vi "Data_get.vi"() -> ()   [LabVIEW 2009]
uses:
  <vilib>/Analysis/2dsp.llb/Real FFT.vi
  <vilib>/Analysis/NI_AALPro.lvlib
panel:
  in  "ps/point":T1(ring)
  in  "ns/div":T2(ring)
  out "Current sweep":u32=1 min=1 max=1000 step=1
  in  "Ext":string="ccd"
  out "Number":string
  in  "Name":string="trace"
  in  "Folder":path
  in  "#Sweeps":u32=1 min=1 max=1000 step=1
  in  "Ampl. (dBm)":dbl min=-135.0 max=30.0 step=0.5 format="%#_8g"
  in  "f (MHz)":dbl=0.0003 min=0.00025 max=67.0 step=1e-06 format="%#.12f"
  in  "Start":bool
  in  "Quit":bool
  in  "E8257D VISA Port":refnum<visa-resource-name>="GPIB0::1::INSTR"
  out "read time (ms)":u32
  out "#points":u32
  out "Busy":bool
  in  "Repetition rate (Hz)":ext=2.5
  in  "Chirp start (MHz)":ext=2.5
  in  "Filter up to (MHz)":ext=2.5
  in  "Amount of averagings":u32=10
  out "Data":dbl[](array[numeric])
  out "XY Graph 5":cluster{ext[], dbl[]}(graph)
  out "FFT (Im)":dbl[](array[numeric])
  out "FFT (Re)":dbl[](array[numeric])
  out "Final array":ext[][](array[numeric])
  out "size(s)":i32
  out "Oscilloscope Data":dbl[](array[numeric])
  in  "Channel Number":u16=1
  out "Oscilloscope graph":dbl[](graph)
  in  "Stop":bool
  in  "TDS VISA Port":refnum<visa-resource-name>="GPIB0::1::INSTR"
  # "TDS6000"
  # "E8257D"
  # "Control"
  # "File Storage"
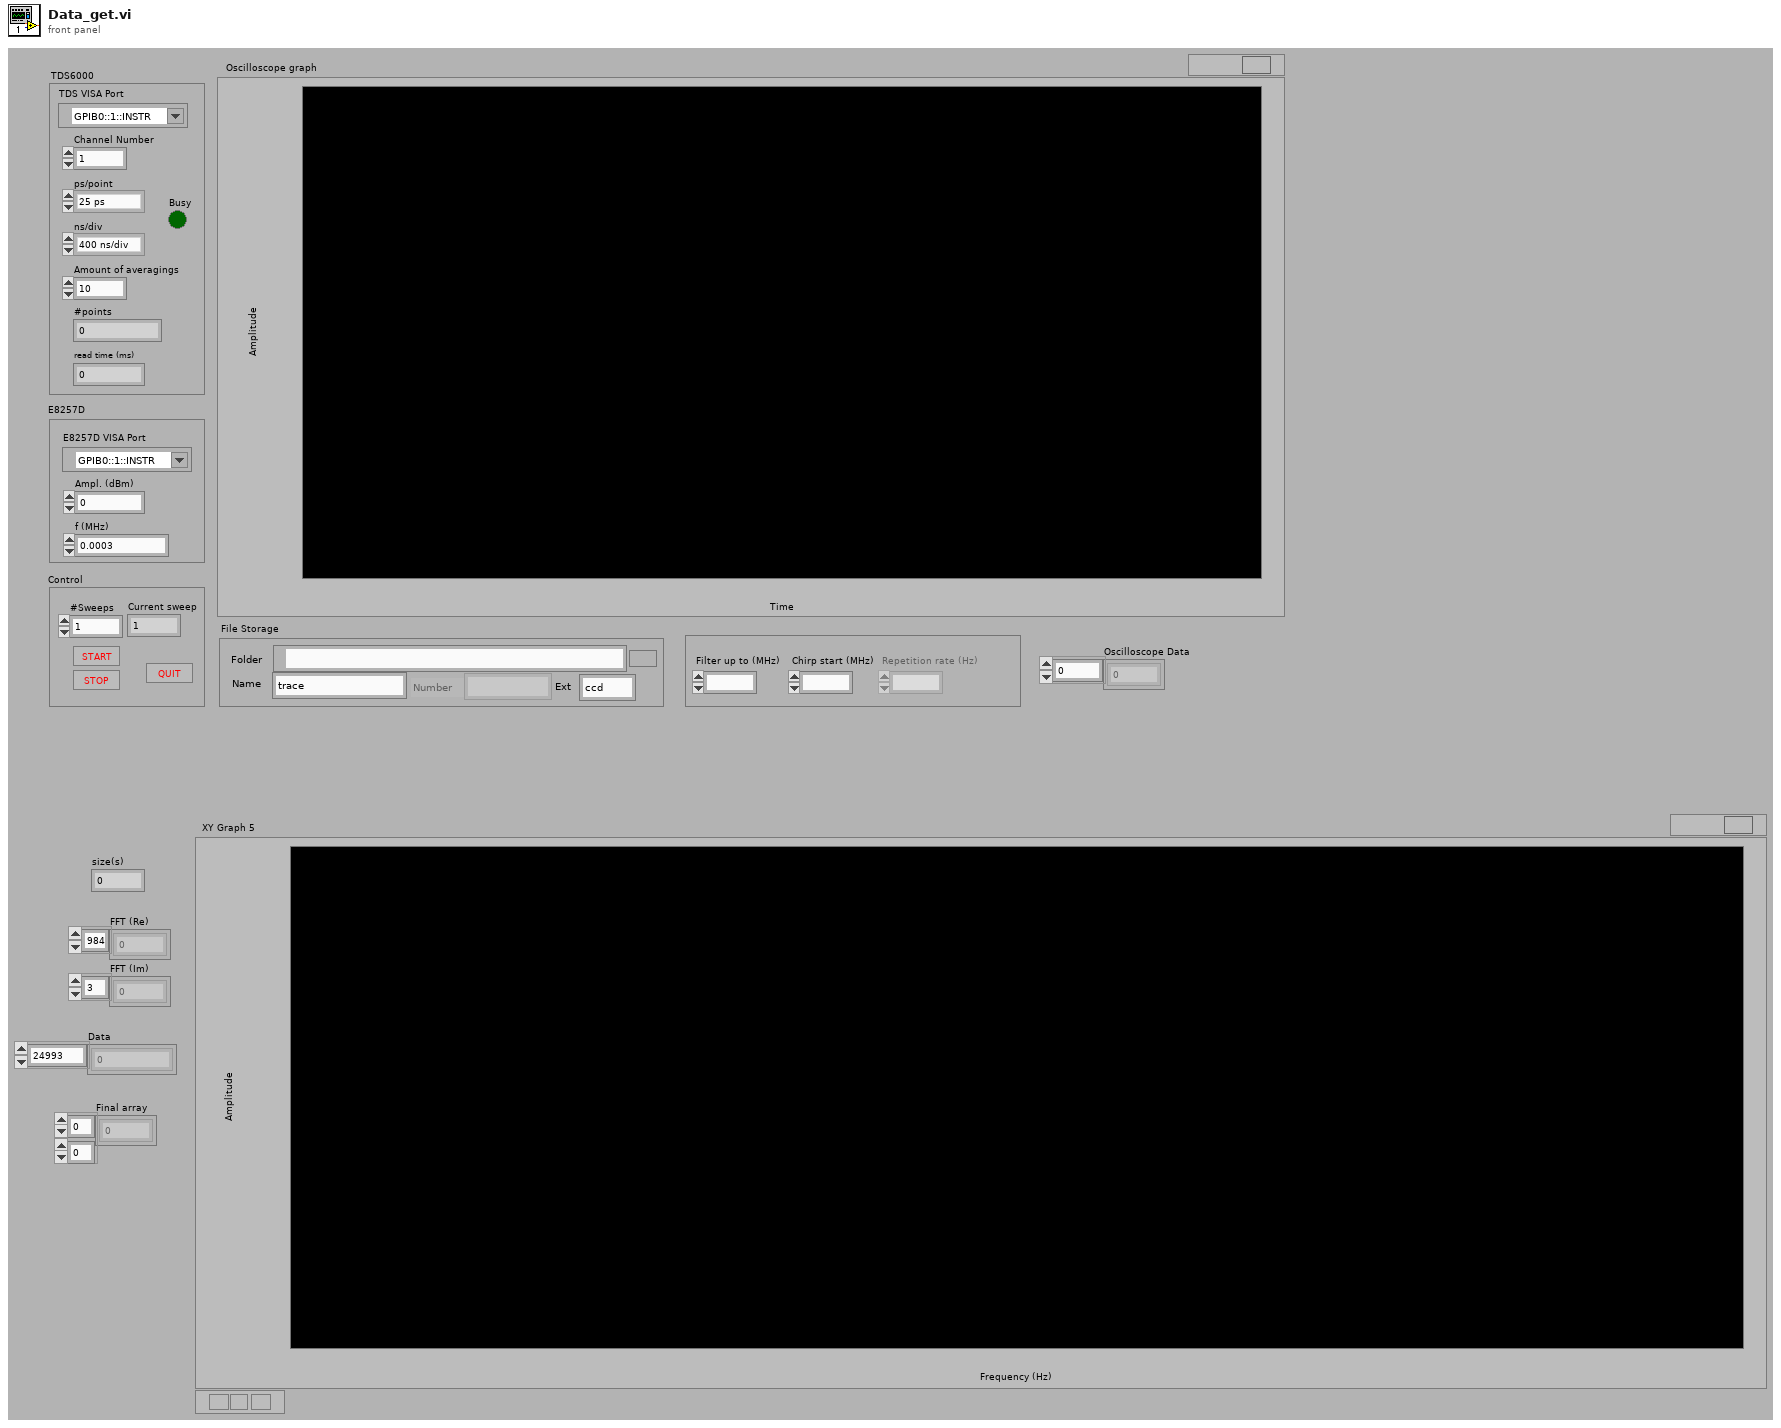
[diagram p1: front panel]
types:
  T1 = enum16{"25 ps", "50 ps", "100 ps", "200 ps", "400 ps", "800 ps", "2 ns"}
  T2 = enum16{"400 ns/div", "1 us/div", "2 us/div", "4 us/div", "10 us/div", "20 us/div"}
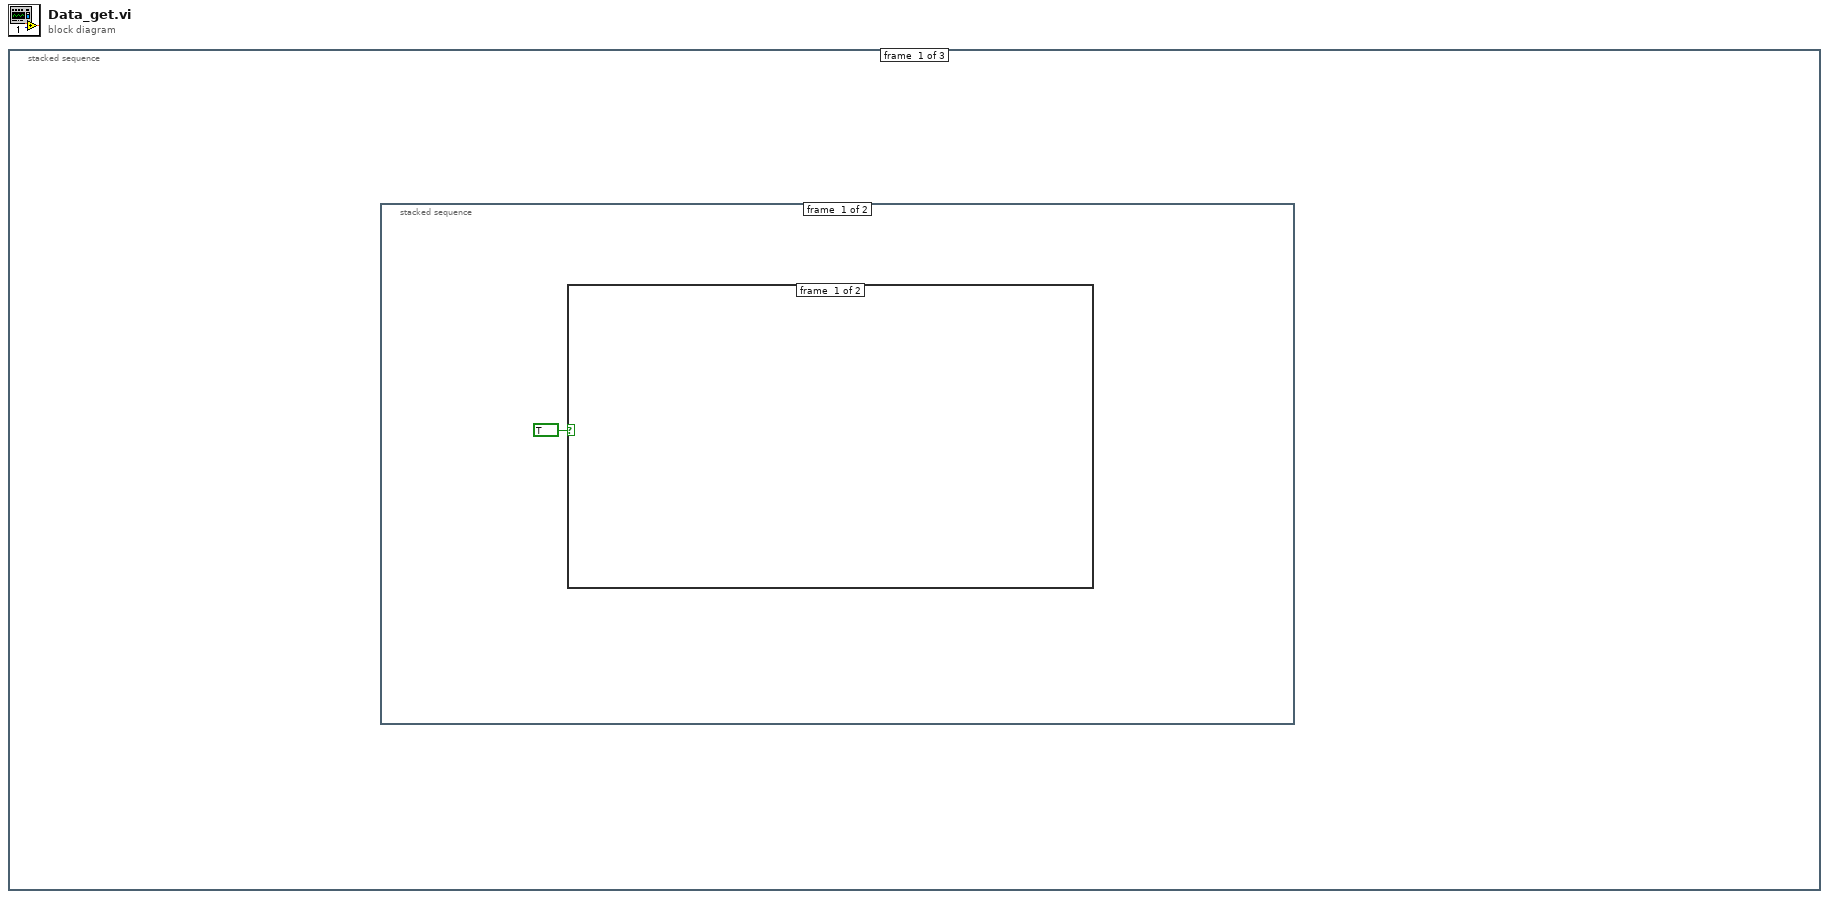
[diagram p0: block diagram]
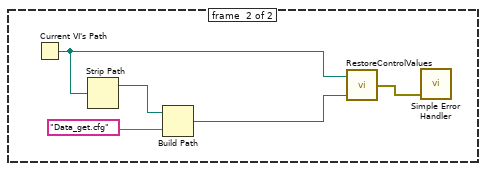
[diagram p2: hidden frame]
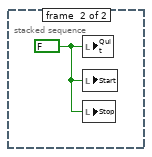
[diagram p3: hidden frame]
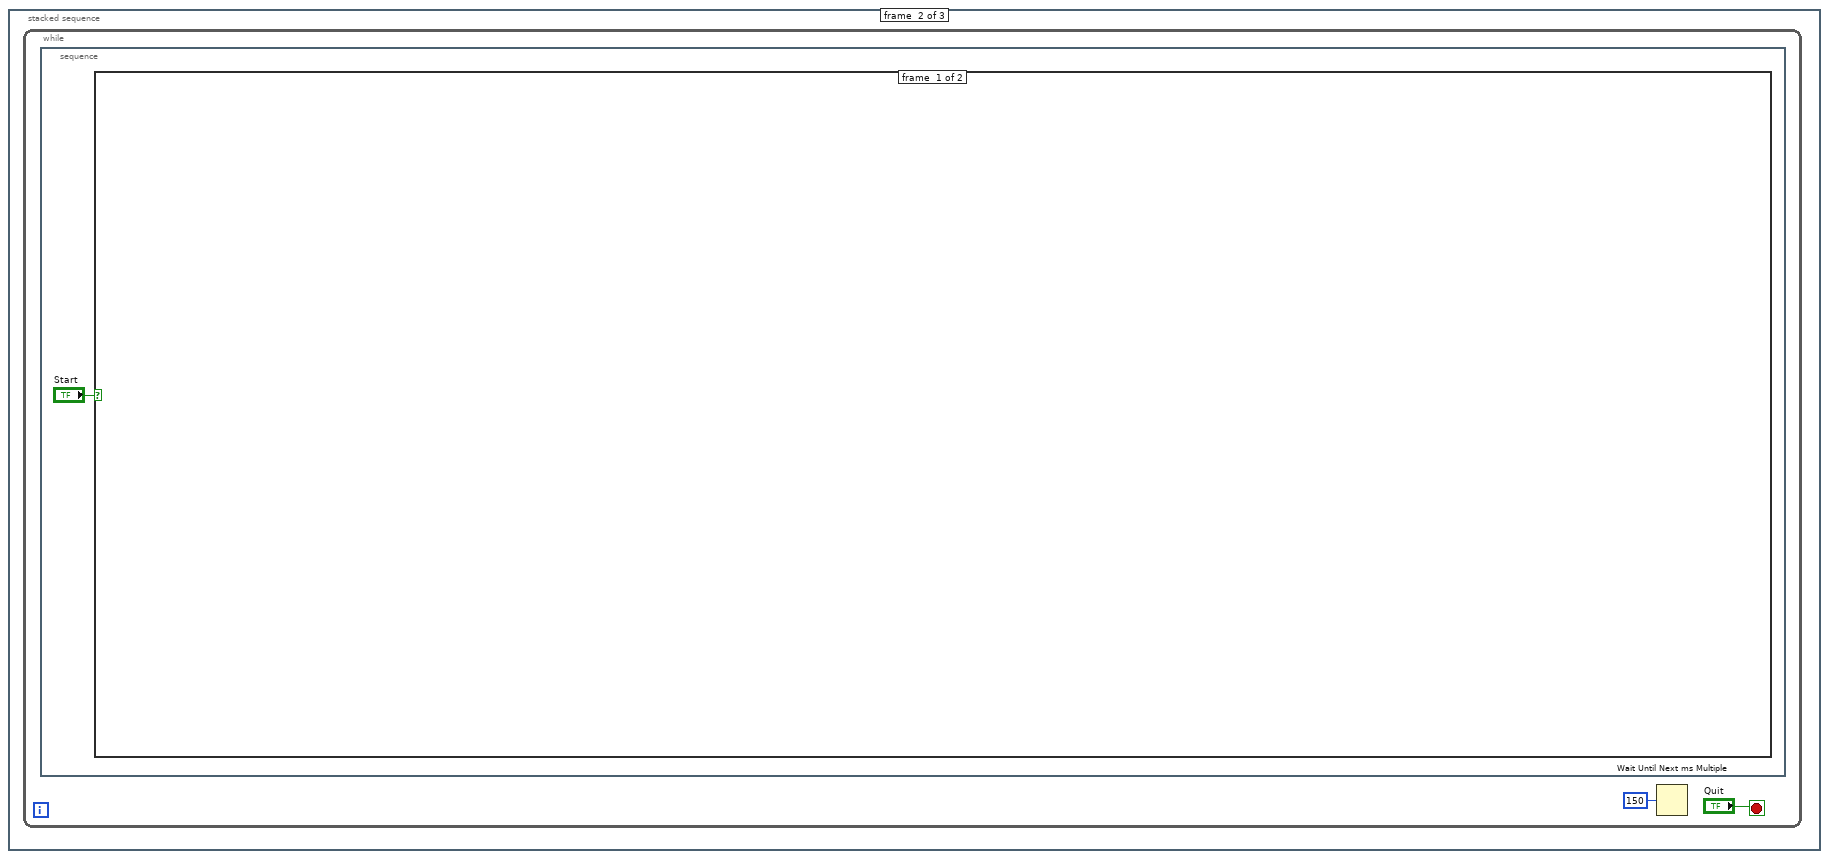
[diagram p4: hidden frame]
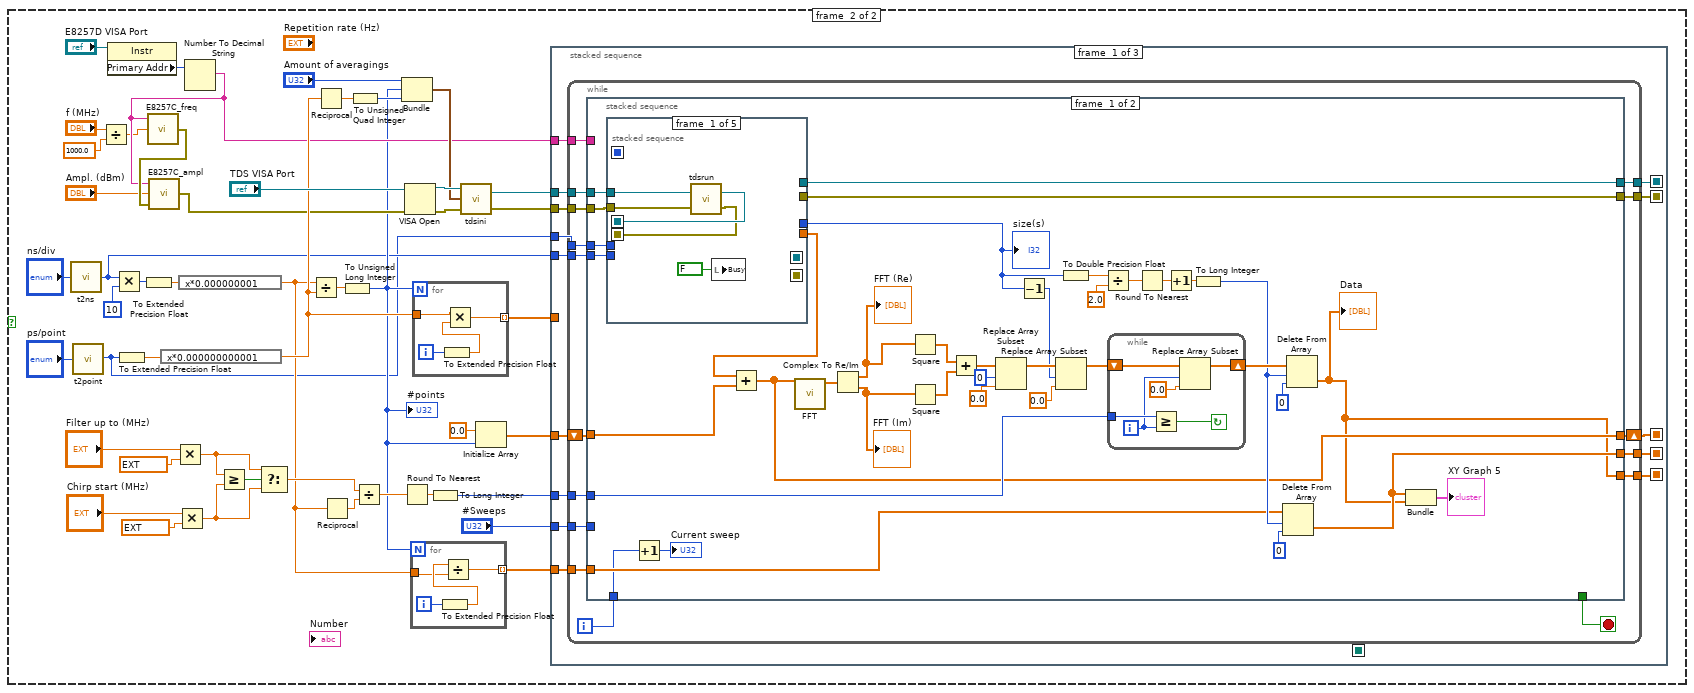
[diagram p5: hidden frame]
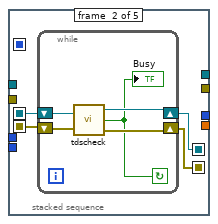
[diagram p6: hidden frame]
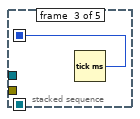
[diagram p7: hidden frame]
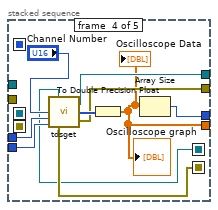
[diagram p8: hidden frame]
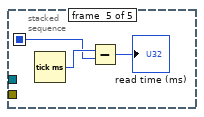
[diagram p9: hidden frame]
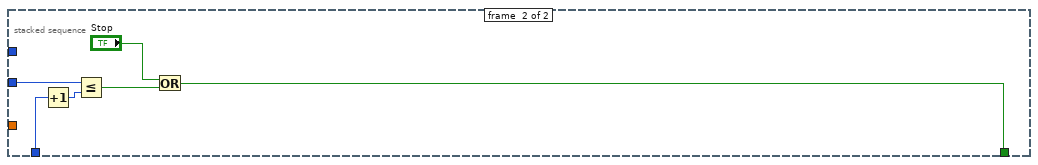
[diagram p10: hidden frame]
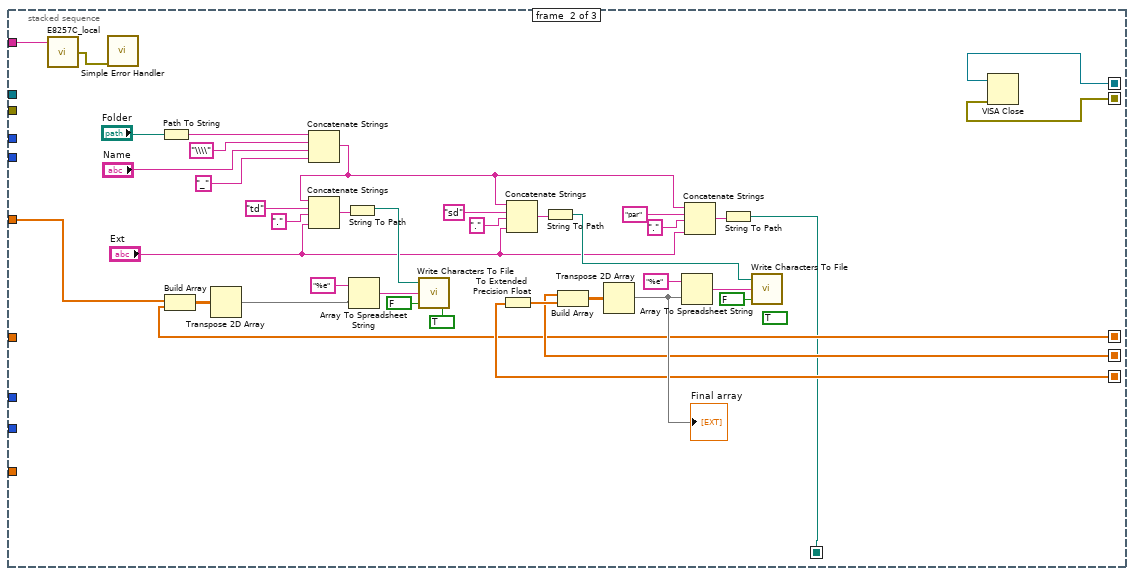
[diagram p11: hidden frame]
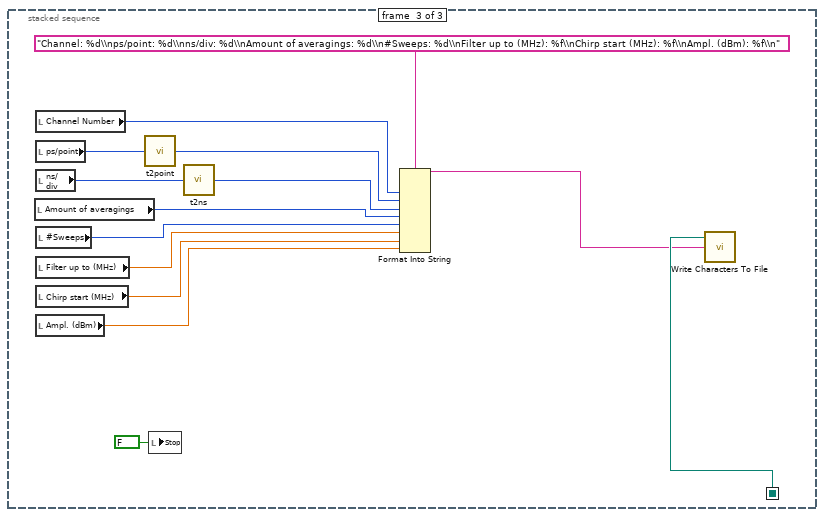
[diagram p12: hidden frame]
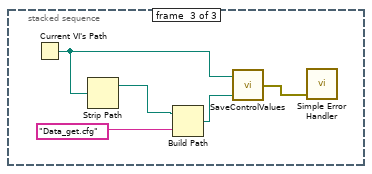
[diagram p13: hidden frame]
diagram:
  n1 = stacked-sequence {
    frame #0 {
      n2 = stacked-sequence {
        frame #0 {
          n3 = case shown="True" TRUE {
            frame #0 {
            }
            frame #1 {
              n4 = Current VI's Path() -> (path=w2:path)
              n5 = Strip Path(path=w2) -> (stripped path=w3:path)  [unwired: 1 out]
              n6 = Build Path(base path=w3, name or relative path="Data_get.cfg") -> (appended path=w5:path)
              n7 = call "RestoreControlValues.vi"("file path"=w5, "vi path"=w2) -> ("error out"=w4:errorcluster)
              n8 = call <vilib>:"Simple Error Handler.vi"("error in (no error)"=w4) -> ()  [unwired: 4 in, 5 out]
            }
          }
        }
        frame #1 {
          w7 = FALSE ("Quit")
          n9 = local write "Quit"(w7) -> ()
          n10 = local write "Start"(w7) -> ()
          n11 = local write "Stop"(w7) -> ()
        }
      }
    }
    frame #1 {
      n12 = while {
        stop <- "Quit" stop-if-true
        n13 = stacked-sequence {
          frame #0 {
            n14 = case shown="True" "Start" {
              frame #0 {
              }
              frame #1 {
                n15 = call "t2ns.vi"("t/div"="ns/div") -> ("ns/div"=w14:u32)
                n16 = call "t2point.vi"("t/point"="ps/point") -> ("ps/point"=w12:u32)
                n17 = Divide(x="f (MHz)", y=1000.0) -> (x/y=w17:dbl)
                n18 = property class="Instr"(reference="E8257D VISA Port") -> ("Primary Addr"=w27:u16)  [unwired: 1 in, 2 out]
                n19 = Multiply(x=w14, y=u32 10) -> (x*y=w51:u32)
                n20 = To Extended Precision Float(1:w12) -> (0:w48:ext)
                n21 = To Extended Precision Float(1:w51) -> (0:w49:ext)
                n22 = expression code="x*0.000000000001"(w48) -> (w33:ext)
                n23 = Multiply(x="Filter up to (MHz)", y=ext 1000000.0) -> (x*y=w39:ext)
                n24 = Multiply(x="Chirp start (MHz)", y=ext 1000000.0) -> (x*y=w36:ext)
                n25 = expression code="x*0.000000001"(w49) -> (w29:ext)
                n26 = Number To Decimal String(number=w27) -> (decimal integer string=w24:string)  [unwired: 1 in]
                n27 = call "E8257C_freq.vi"("Frequency GHz"=w17, "GPIB address"=w24) -> ("error out"=w25:errorcluster)  [unwired: 1 in]
                n28 = call "E8257C_ampl.vi"("error in"=w25, "Amplitude dBm"="Ampl. (dBm)", "GPIB address"=w24) -> ("error out"=w23:errorcluster)
                n29 = Greater Or Equal?(x=w39, y=w36) -> (x >= y?=w47:bool)
                n30 = Select(t=w39, s=w47, f=w36) -> (s? t:f=w45:ext)
                n31 = Divide(x=w29, y=w33) -> (x/y=w50:ext)
                n32 = Reciprocal(x=w33) -> (1/x=w31:ext)
                n33 = Reciprocal(x=w29) -> (1/x=w46:ext)
                n34 = To Unsigned Long Integer(number=w50) -> (unsigned 32bit integer=w19:u32)
                "#points" <- w19
                n35 = To Unsigned Quad Integer(1:w31) -> (0:w32:u64)
                n36 = Divide(x=w45, y=w46) -> (x/y=w44:ext)
                n37 = Bundle("Amount of averagings"="Amount of averagings", w19, w32) -> (w34:cluster{"Amount of averagings ":u32, u32, u64})  [unwired: 1 in]
                n38 = Round To Nearest(number=w44) -> (nearest integer value=w43:ext)
                n39 = VISA Open(error in (no error)=w23, VISA resource name="TDS VISA Port") -> (VISA resource name=w54:refnum<visa-resource-name>, error out=w55:errorcluster)  [unwired: 3 in]
                n40 = for {
                  N: w19 -> [_]
                  tunnel: w29 -> [w219]
                  tunnel: [w221] -> w30 mode=indexing
                  i -> [w222]
                  n41 = To Extended Precision Float(1:w222) -> (0:w220:ext)
                  n42 = Divide(x=w220, y=w219) -> (x/y=w221:ext)
                }
                n43 = for {
                  N: w19 -> [_]
                  tunnel: w33 -> [w224]
                  tunnel: [w223] -> w15 mode=indexing
                  i -> [w226]
                  n44 = To Extended Precision Float(1:w226) -> (0:w225:ext)
                  n45 = Multiply(x=w224, y=w225) -> (x*y=w223:ext)
                }
                n46 = To Long Integer(number=w43) -> (32bit integer=w42:i32)
                n47 = call "tdsini.vi"("Error In (No Error)"=w55, "Acq_par"=w34, "VISA Port In"=w54) -> ("Error Out"=w56:errorcluster, "VISA Port Out"=w57:refnum<visa-resource-name>)
                n48 = Initialize Array(0.0 ("element"), w19) -> (w18:dbl[])
                n49 = stacked-sequence {
                  seq-local: [w62 _ _] -> [_ w204 _]
                  seq-local: [w61 _ _] -> [_ w203 _]
                  seq-local: [w60 _ _] -> [_ w191 _]
                  seq-local: [w59 _ _] -> [_ w194 _]
                  seq-local: [w58 _ _] -> [_ w193 _]
                  seq-local: [_ w167 _] -> [_ _ w218]
                  tunnel: w57 -> [w71 _ _]
                  tunnel: w56 -> [w70 _ _]
                  tunnel: w12 -> [w69 _ _]
                  tunnel: w14 -> [w68 _ _]
                  tunnel: w42 -> [w67 _ _]
                  tunnel: w30 -> [w66 _ _]
                  tunnel: w24 -> [w65 w201 _]
                  tunnel: "#Sweeps" -> [w64 _ _]
                  tunnel: w18 -> [w63 _ _]
                  tunnel: w15 -> [_ w166 _]
                  frame #0 {
                    n50 = while {
                      tunnel: [w84] -> w61
                      tunnel: [w85] -> w62
                      tunnel: w70 -> [w86]
                      tunnel: w71 -> [w87]
                      tunnel: w69 -> [w83]
                      tunnel: w68 -> [w82]
                      tunnel: w66 -> [w80]
                      tunnel: w67 -> [w81]
                      tunnel: w65 -> [w77]
                      tunnel: w64 -> [w76]
                      shift-right: [w74] -> w60
                      shift-left: w63 -> [w75]
                      tunnel: [w73] -> w59
                      tunnel: [w72] -> w58
                      i -> [w79]
                      stop <- w78 stop-if-true
                      n51 = stacked-sequence {
                        tunnel: w87 -> [w125 _]
                        tunnel: w86 -> [w124 _]
                        tunnel: [w123 _] -> w85
                        tunnel: [w122 _] -> w84
                        tunnel: w83 -> [w121 _]
                        tunnel: w82 -> [w120 _]
                        tunnel: w81 -> [w106 _]
                        tunnel: w80 -> [w95 _]
                        tunnel: w79 -> [w88 w165]
                        tunnel: [_ w162] -> w78
                        tunnel: w77 -> [_ _]
                        tunnel: w76 -> [_ w161]
                        tunnel: w75 -> [w94 _]
                        tunnel: [w92 _] -> w74
                        tunnel: [w91 _] -> w73
                        tunnel: [w90 _] -> w72
                        frame #0 {
                          n52 = stacked-sequence {
                            seq-local: [w134 _ _ _ _] -> [_ w140 _ _ _]
                            seq-local: [w133 _ _ _ _] -> [_ w139 _ _ _]
                            seq-local: [_ w137 _ _ _] -> [_ _ _ w148 _]
                            seq-local: [_ w138 _ _ _] -> [_ _ _ w147 _]
                            seq-local: [_ _ w146 _ _] -> [_ _ _ _ w158]
                            tunnel: w125 -> [w135 _ _ _ _]
                            tunnel: w124 -> [w136 _ _ _ _]
                            tunnel: [_ _ _ w155 _] -> w123
                            tunnel: [_ _ _ w154 _] -> w122
                            tunnel: w121 -> [_ _ _ w152 _]
                            tunnel: w120 -> [_ _ _ w151 _]
                            tunnel: [_ _ _ w150 _] -> w104
                            tunnel: [_ _ _ w149 _] -> w93
                            frame #0 {
                              n53 = call "tdsrun.vi"("Error In (No Error)"=w136, "VISA Port In"=w135) -> ("Error Out"=w133:errorcluster, "VISA Port Out"=w134:refnum<visa-resource-name>)
                              n54 = local write "Busy"(FALSE ("Busy")) -> ()
                            }
                            frame #1 {
                              n55 = while {
                                shift-right: [w143] -> w138
                                shift-left: w140 -> [w144]
                                shift-right: [w142] -> w137
                                shift-left: w139 -> [w145]
                                stop <- w141 continue-if-true
                                n56 = call "tdscheck.vi"("VISA Port In"=w144, "Error In (No Error)"=w145) -> ("VISA Port Out"=w143:refnum<visa-resource-name>, "busy"=w141:bool, "Error Out"=w142:errorcluster)
                                "Busy" <- w141
                              }
                            }
                            frame #2 {
                              n57 = Tick Count (ms)() -> (millisecond timer value=w146:u32)
                            }
                            frame #3 {
                              n58 = call "tdsget.vi"("VISA Port In"=w147, "Channel Number"="Channel Number", "ps/point"=w152, "ns/div"=w151, "Error In (No Error)"=w148) -> ("VISA Port Out"=w155:refnum<visa-resource-name>, "TDS Data"=w156:u16[], "Error Out"=w154:errorcluster)  [unwired: 8 in]
                              n59 = To Double Precision Float(number=w156) -> (double precision float=w149:dbl[])
                              "Oscilloscope graph" <- w149
                              "Oscilloscope Data" <- w149
                              n60 = Array Size(array=w149) -> (size(s)=w150:i32)
                            }
                            frame #4 {
                              n61 = Tick Count (ms)() -> (millisecond timer value=w159:u32)
                              n62 = Subtract(x=w159, y=w158) -> (x-y=→"read time (ms)":u32)
                            }
                          }
                          "size(s)" <- w104
                          n63 = Increment(x=w88) -> (x+1=→"Current sweep":i32)
                          n64 = Add(x=w93, y=w94) -> (x+y=w92:dbl[])
                          n65 = call-poly <vilib>:"FFT.vi"("X"=w92) -> ("FFT {X}"=w119:cdb[])  [unwired: 9 in, 1 out]
                          n66 = Complex To Re/Im(x + iy=w119) -> (x=w118:dbl[], y=w117:dbl[])
                          "FFT (Re)" <- w118
                          "FFT (Im)" <- w117
                          n67 = Square(x=w118) -> (x^2=w116:dbl[])
                          n68 = Square(x=w117) -> (x^2=w115:dbl[])
                          n69 = Add(x=w116, y=w115) -> (x+y=w111:dbl[])
                          n70 = Replace Array Subset(array=w111, new element=0.0 ("new element/subarray"), index=0) -> (w110:dbl[])
                          n71 = Decrement(x=w104) -> (x-1=w109:i32)
                          n72 = Replace Array Subset(array=w110, new element=0.0 ("new element/subarray"), index=w109) -> (w107:dbl[])
                          n73 = To Double Precision Float(number=w104) -> (double precision float=w103:dbl)
                          n74 = Divide(x=w103, y=2.0) -> (x/y=w101:dbl)
                          n75 = while {
                            tunnel: w106 -> [w130]
                            shift-right: [w128] -> w105
                            shift-left: w107 -> [w129]
                            i -> [w127]
                            stop <- w131 continue-if-true
                            n76 = Greater Or Equal?(x=w130, y=w127) -> (x >= y?=w131:bool)
                            n77 = Replace Array Subset(array=w129, new element=0.0 ("new element/subarray"), index=w127) -> (w128:dbl[])
                          }
                          n78 = Round To Nearest(number=w101) -> (nearest integer value=w100:dbl)
                          n79 = Increment(x=w100) -> (x+1=w99:dbl)
                          n80 = To Long Integer(number=w99) -> (32bit integer=w96:i32)
                          n81 = Delete From Array(array=w95, length=w96, index=0) -> (deleted portion=w91:ext[])  [unwired: 1 out]
                          n82 = Delete From Array(array=w105, length=w96, index=0) -> (deleted portion=w90:dbl[])  [unwired: 1 out]
                          "Data" <- w90
                          n83 = Bundle(w91, w90) -> (→"XY Graph 5":cluster{ext[], dbl[]})  [unwired: 1 in]
                        }
                        frame #1 {
                          n84 = Increment(x=w165) -> (x+1=w160:i32)
                          n85 = Less Or Equal?(x=w161, y=w160) -> (x <= y?=w164:bool)
                          n86 = Or(x="Stop", y=w164) -> (x .or. y?=w162:bool)
                        }
                      }
                    }
                  }
                  frame #1 {
                    (unwired) TRUE
                    n87 = call "E8257C_local.vi"("GPIB address"=w201) -> ("error out"=w202:errorcluster)  [unwired: 1 in]
                    n88 = call <vilib>:"Simple Error Handler.vi"("error in (no error)"=w202) -> ()  [unwired: 4 in, 5 out]
                    n89 = Path To String(path="Folder") -> (string=w190:string)
                    n90 = Build Array(w166, w191) -> (w192:ext[][])
                    n91 = Transpose 2D Array(2D array=w192) -> (transposed array=w177:ext[][])
                    n92 = Concatenate Strings(w190, "\\\\" ("string"), "Name", "_") -> (w169:string)
                    n93 = Concatenate Strings(w169, "td", ".", "Ext") -> (w183:string)
                    n94 = String To Path(string=w183) -> (path=w178:path)
                    n95 = Array To Spreadsheet String(array=w177, 3:"%e") -> (spreadsheet string=w180:string)  [unwired: 1 in]
                    n96 = call <vilib>:"Write Characters To File.vi"("convert eol? (no:F)"=TRUE, "append to file? (new file:F)"=FALSE, "character string"=w180, "file path (dialog if empty)"=w178) -> ()  [unwired: 1 in, 1 out]
                    n97 = To Extended Precision Float(1:w193) -> (0:w195:ext[])
                    n98 = Concatenate Strings(w169, "sd", ".", "Ext") -> (w174:string)
                    n99 = String To Path(string=w174) -> (path=w173:path)
                    n100 = Build Array(w194, w195) -> (w196:ext[][])
                    n101 = Transpose 2D Array(2D array=w196) -> (transposed array=w199:ext[][])
                    "Final array" <- w199
                    n102 = Array To Spreadsheet String(array=w199, 3:"%e") -> (spreadsheet string=w197:string)  [unwired: 1 in]
                    n103 = Concatenate Strings(w169, "par", ".", "Ext") -> (w170:string)
                    n104 = String To Path(string=w170) -> (path=w167:path)
                    n105 = call <vilib>:"Write Characters To File.vi"("append to file? (new file:F)"=FALSE, "character string"=w197, "file path (dialog if empty)"=w173) -> ()  [unwired: 2 in, 1 out]
                    n106 = VISA Close(VISA resource name=w204, error in (no error)=w203) -> ()  [unwired: 1 out]
                  }
                  frame #2 {
                    n107 = local read "Amount of averagings"() -> (w212:u32)
                    n108 = local read "Channel Number"() -> (w215:u16)
                    n109 = local read "ps/point"() -> (w214:T1)
                    n110 = local read "ns/div"() -> (w213:T2)
                    n111 = local read "#Sweeps"() -> (w210:u32)
                    n112 = local read "Filter up to (MHz)"() -> (w209:ext)
                    n113 = local read "Chirp start (MHz)"() -> (w208:ext)
                    n114 = local read "Ampl. (dBm)"() -> (w207:dbl)
                    n115 = call "t2point.vi"("t/point"=w214) -> ("ps/point"=w205:u32)
                    n116 = local write "Stop"(FALSE ("Stop")) -> ()
                    n117 = call "t2ns.vi"("t/div"=w213) -> ("ns/div"=w206:u32)
                    n118 = Format Into String(format string="Channel: %d\\nps/point: %d\\nns/div: %d\\nAmount of averagings: %d\\n#Sweeps: %d\\nFilter up to (MHz): %f\\nChirp start (MHz): %f\\nAmpl. (dBm): %f\\n", w215, w205, w206, w212, w210, w209, w208, w207) -> (resulting string=w217:string)  [unwired: 2 in, 1 out]
                    n119 = call <vilib>:"Write Characters To File.vi"("character string"=w217, "file path (dialog if empty)"=w218) -> ()  [unwired: 3 in, 1 out]
                  }
                }
              }
            }
          }
        }
        n120 = Wait Until Next ms Multiple(millisecond multiple=u32 150) -> ()  [unwired: 1 out]
      }
    }
    frame #2 {
      n121 = Current VI's Path() -> (path=w227:path)
      n122 = Strip Path(path=w227) -> (stripped path=w228:path)  [unwired: 1 out]
      n123 = Build Path(base path=w228, name or relative path="Data_get.cfg") -> (appended path=w230:path)
      n124 = call "SaveControlValues.vi"("file path"=w230, "vi path"=w227) -> ("error out"=w229:errorcluster)
      n125 = call <vilib>:"Simple Error Handler.vi"("error in (no error)"=w229) -> ()  [unwired: 4 in, 5 out]
    }
  }
